vi "Signed Array Index.vi"(9 "Array Size":i32, 10 "Array Index in":i32) -> (1 "Out of Range?":bool, 2 "Array Index out":i32)   [LabVIEW 2019]
doc: "Converts negative index i (i.e. starting from array end) to regular index.\n-1: last element, etc.\nIf i > n or i < -n - 1, where n + 1 is the array size, the result is the default LabVIEW output for an out of bound index value."
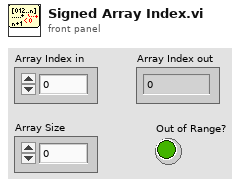
[diagram p1: front panel]
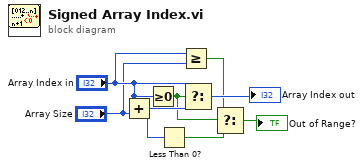
[diagram p0: block diagram]
diagram:
  n1 = Add(x="Array Index in", y="Array Size") -> (x+y=w5:i32)
  n2 = Greater Or Equal To 0?(x="Array Index in") -> (x >= 0?=w4:bool)
  n3 = Less Than 0?(x=w5) -> (x < 0?=w2:bool)
  n4 = Greater Or Equal?(x="Array Index in", y="Array Size") -> (x >= y?=w3:bool)
  n5 = Select(t="Array Index in", s=w4, f=w5) -> (s? t:f=→"Array Index out":i32)
  n6 = Select(t=w3, s=w4, f=w2) -> (s? t:f=→"Out of Range?":bool)
